vi "Launcher.vi"() -> ()   [LabVIEW 2015]
uses:
  Money/Money.lvlib
panel:
  in  "Hide Panel":bool
  in  "Show Panel":bool
  in  "Stop Button":bool
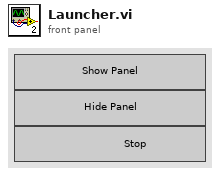
[diagram p1: front panel]
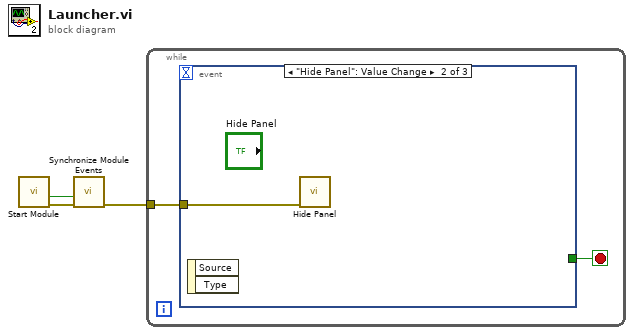
[diagram p0: block diagram]
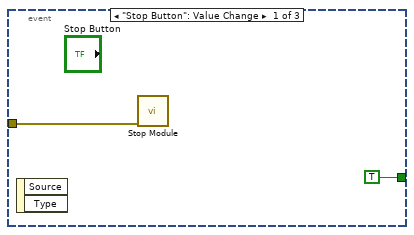
[diagram p2: hidden frame]
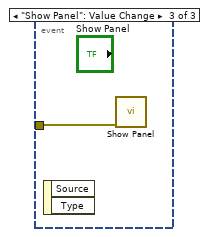
[diagram p3: hidden frame]
diagram:
  n1 = call "Start Module.vi"() -> ("error out"=w1:errorcluster, "Wait for Event Sync?"=w3:bool)  [unwired: 8 in, 2 out]
  n2 = call "Synchronize Module Events.vi"("error in (no error)"=w1, "Wait for Event Sync?"=w3) -> ("error out"=w2:errorcluster)  [unwired: 9 in]
  n3 = while {
    tunnel: w2 -> [w5]
    stop <- w4 stop-if-true
    n4 = event shown="[1] \"Hide Panel\": Value Change" {
      selector: _ -> [_ _ _]
      dyn-events: _ -> [_ _ _]
      timeout: _ -> [_ _ _]
      tunnel: w5 -> [w6 w8 w9]
      tunnel: [TRUE _ _] -> w4
      event "Stop Button": Value Change {
        n5 = event-data() -> ()  [unwired: 1 in, 2 out]
        n6 = call "Stop Module.vi"("error in (no error)"=w6) -> ()  [unwired: 10 in, 1 out]
      }
      event "Hide Panel": Value Change {
        n7 = event-data() -> ()  [unwired: 1 in, 2 out]
        n8 = call "Hide Panel.vi"("error in (no error)"=w8) -> ()  [unwired: 10 in, 1 out]
      }
      event "Show Panel": Value Change {
        n9 = event-data() -> ()  [unwired: 1 in, 2 out]
        n10 = call "Show Panel.vi"("error in (no error)"=w9) -> ()  [unwired: 10 in, 1 out]
      }
    }
  }
